vi "Disconnect.vi"(0 "reference in":refnum<class "Switch_2739.lvclass">, 1 "channel 1":string, 2 "channel 2":string, 5 "error in (no error)":errorcluster) -> (14 "reference in":refnum<class "Switch_2739.lvclass">, 19 "error out":errorcluster)   [LabVIEW 2017]
uses:
  Switch_2739.lvclass
  <userlib>/_OpenG.lib/string/string.llb/Trim Whitespace (String)__ogtk.vi
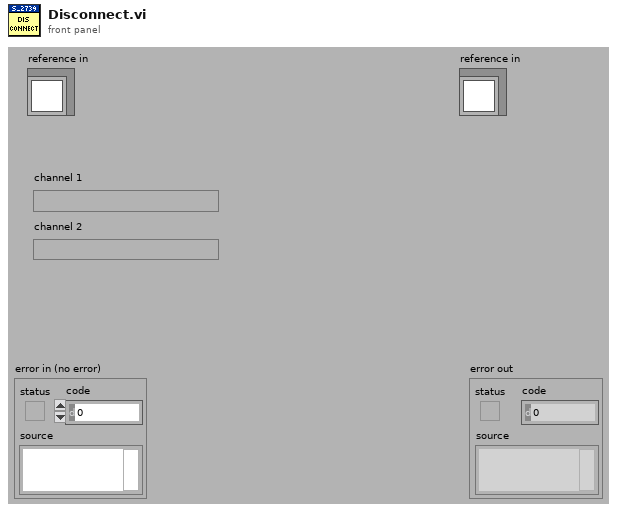
[diagram p1: front panel]
types:
  T1 = typedef "Switch_2739.lvlib/Switch_2739.lvclass/ObjectAttributes.ctl" = cluster{"Config":T2, "MatrixState":bool[][]}
  T2 = typedef "Switch_2739.lvlib/Switch_2739.lvclass/Config.ctl" = cluster{"Resource":refnum<k15>, "SwitchMap":cluster{"Name":string, "Route":string[][]}[]}
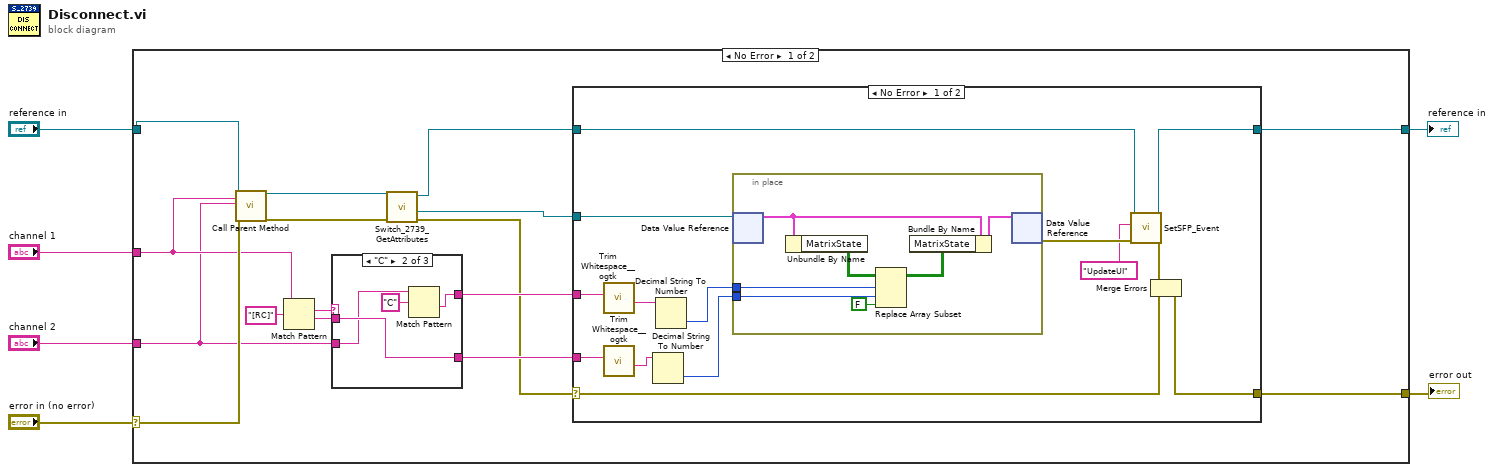
[diagram p0: block diagram]
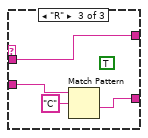
[diagram p3: hidden frame]
diagram:
  n1 = case shown="No Error" "error in (no error)" {
    selector: "error in (no error)" -> [w21 w55]
    tunnel: [w10 w55] -> w5
    tunnel: [w11 w54] -> w3
    tunnel: "reference in" -> [w22 w54]
    tunnel: "channel 2" -> [w7 _]
    tunnel: "channel 1" -> [w8 _]
    frame No Error {
      n2 = call-parent "Call Parent Method"("reference in"=w22, "channel 1"=w8, 2:w7, "error in (no error)"=w21) -> ("reference in"=w13:refnum<class "Switch_2739.lvclass">, "error out"=w12:errorcluster)  [unwired: 14 in]
      n3 = Match Pattern(string=w8, regular expression="[RC]") -> (match substring=w18:string, after substring=w17:string)  [unwired: 1 in, 2 out]
      n4 = case shown="\"C\"" w18 {
        tunnel: w17 -> [_ w26 w30]
        tunnel: [_ w23 w30] -> w16
        tunnel: w7 -> [_ w24 w28]
        tunnel: [_ w26 w27] -> w15
        frame Default {
        }
        frame "C" {
          n5 = Match Pattern(string=w24, regular expression="C") -> (after substring=w23:string)  [unwired: 1 in, 3 out]
        }
        frame "R" {
          (unwired) TRUE
          n6 = Match Pattern(string=w28, regular expression="C") -> (after substring=w27:string)  [unwired: 1 in, 3 out]
        }
      }
      n7 = call "Switch_2739_GetAttributes.vi"("error in (no error)"=w12, "reference in"=w13) -> ("error out"=w14:errorcluster, "DataRef"=w20:refnum<data-value>, "reference out"=w19:refnum<class "Switch_2739.lvclass">)  [unwired: 6 in, 1 out]
      n8 = case shown="No Error" w14 {
        selector: w14 -> [w31 w52]
        tunnel: w20 -> [w44 _]
        tunnel: w19 -> [w43 w53]
        tunnel: [w42 w53] -> w11
        tunnel: [w39 w52] -> w10
        tunnel: w16 -> [w37 _]
        tunnel: w15 -> [w36 _]
        frame No Error {
          n9 = call-poly <userlib>:"Trim Whitespace__ogtk.vi"("String in"=w37) -> ("String out"=w35:string)  [unwired: 6 in]
          n10 = call-poly <userlib>:"Trim Whitespace__ogtk.vi"("String in"=w36) -> ("String out"=w34:string)  [unwired: 6 in]
          n11 = Decimal String To Number(string=w34) -> (number=w32:i32)  [unwired: 2 in, 1 out]
          n12 = Decimal String To Number(string=w35) -> (number=w33:i32)  [unwired: 2 in, 1 out]
          n13 = in-place {
            in-place-border: w33 -> [w50]
            in-place-border: w32 -> [w49]
            n14 = in-place-dvr #1(w44) -> (w47:T1)  [unwired: 1 out]
            n15 = Unbundle By Name(w47) -> ("MatrixState"=w51:bool[][])
            n16 = Replace Array Subset(array=w51, new element=FALSE ("new element/subarray"), index (row)=w50, index (col)=w49) -> (w46:bool[][])
            n17 = Bundle By Name(cluster=w47, "MatrixState"=w46) -> (w45:T1)
            n18 = in-place-dvr #1(w45) -> (w41:errorcluster)  [unwired: 1 out]
          }
          n19 = call-dynamic "SetSFP_Event.vi"("error in (no error)"=w41, "msg"="UpdateUI", "reference in"=w43) -> ("error out"=w40:errorcluster, "reference out"=w42:refnum<class "Switch_2739.lvclass">)  [unwired: 7 in]
          n20 = Merge Errors(w40, w31) -> (w39:errorcluster)
        }
        frame Error {
        }
      }
    }
    frame Error {
    }
  }
  "error out" <- w5
  "reference in" <- w3
